vi "1D Quadrature Formula Str Func.vi"(10 "data":variant, 11 "X":dbl[](array[numeric])) -> (0 "error out":errorcluster, 3 "F(X)":dbl[](array[numeric]))   [LabVIEW 2014, in "NI_AALPro.lvlib"]
uses:
  NI_AALPro.lvlib
  NI_Gmath.lvlib
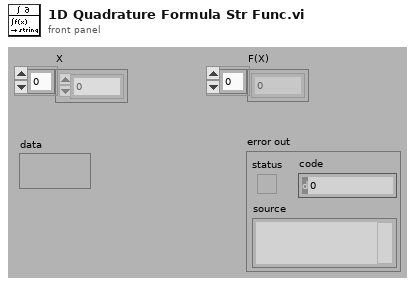
[diagram p1: front panel]
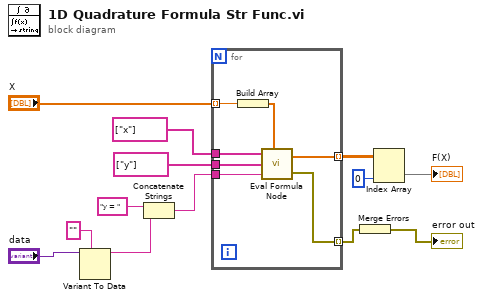
[diagram p0: block diagram]
diagram:
  n1 = Variant To Data(type="" ("string"), Variant="data") -> (data=w6:string)  [unwired: 1 in, 1 out]
  n2 = Concatenate Strings("y = " ("string"), w6) -> (w12:string)
  n3 = for {
    tunnel: w12 -> [w20]
    tunnel: string[] ["y"] ("Variables Output") -> [w19]
    tunnel: string[] ["x"] ("Variables Output") -> [w18]
    tunnel: "X" -> [w17] mode=indexing
    tunnel: [w15] -> w3 mode=indexing
    tunnel: [w14] -> w4 mode=indexing
    n4 = Build Array(w17) -> (w16:dbl[])
    n5 = call "Eval Formula Node.vi"("Variables Input"=w18, "Input Values"=w16, "Variables Output"=w19, "formula"=w20) -> ("Output Values"=w15:dbl[], "error out"=w14:errorcluster)  [unwired: 1 in]
  }
  n6 = Merge Errors(w4) -> (→"error out":errorcluster)
  n7 = Index Array(array=w3, index (col)=0 ("disabled index (col)")) -> (element=→"F(X)":dbl[])  [unwired: 1 in]
